vi "Message Buffer.vi"(6 "Reset":bool, 8 "postdata":string, 9 "Data":string, 10 "UID":string, 11 "Command":string) -> (3 "Personnel Posts":string[](array[string]))   [LabVIEW 2015]
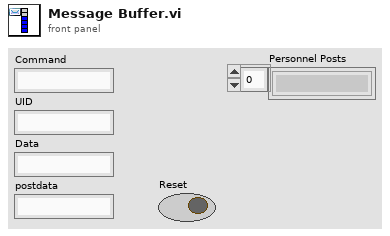
[diagram p1: front panel]
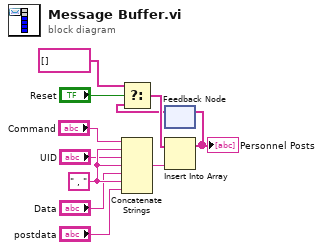
[diagram p0: block diagram]
diagram:
  w11 = " , " ("string")
  n1 = Concatenate Strings("Command", w11, "UID", w11, "Data", w11, "postdata") -> (w5:string)
  n2 = feedback #1() -> (w8:string[])  [unwired: 1 in]
  n3 = Select(t=string[] [], s="Reset", f=w8) -> (s? t:f=w10:string[])
  n4 = Insert Into Array(array=w10, new element=w5) -> (w6:string[])  [unwired: 1 in]
  "Personnel Posts" <- w6
  n5 = feedback-in #1(w6) -> ()
